vi "Crop Rotate Resize to U16.vi"() -> ()   [LabVIEW 2023]
uses:
  <vilib>/vision/NI_Vision_Development_Module.lvlib
panel:
  in  "2nd Resample":bool
  in  "2nd crop":bool
  in  "Symmetry":bool
  in  "Type of Symmetry":u32(ring)=1 items=["Horizontal", "Vertical", "Central", "1st Diagonal", "2nd Diagonal"]
  out "Image 3":T1(plugin-control)
  in  "Maintain Size":bool
  in  "resize":bool=TRUE
  in  "Do it":bool
  in  "stop":bool
  in  "Invert":bool
  in  "X Resolution":i32=1024
  in  "Y Resolution":i32=1024
  in  "Angle (degrees)":dbl format="%#_13g"
  in  "Destination File Path":path
  in  "Source File Path":path
  out "Image 2":T1(plugin-control)
  out "Image":T1(plugin-control)
  # "Nothing special, just my very internal VI to Crop/Resize/Rotate images if needed"
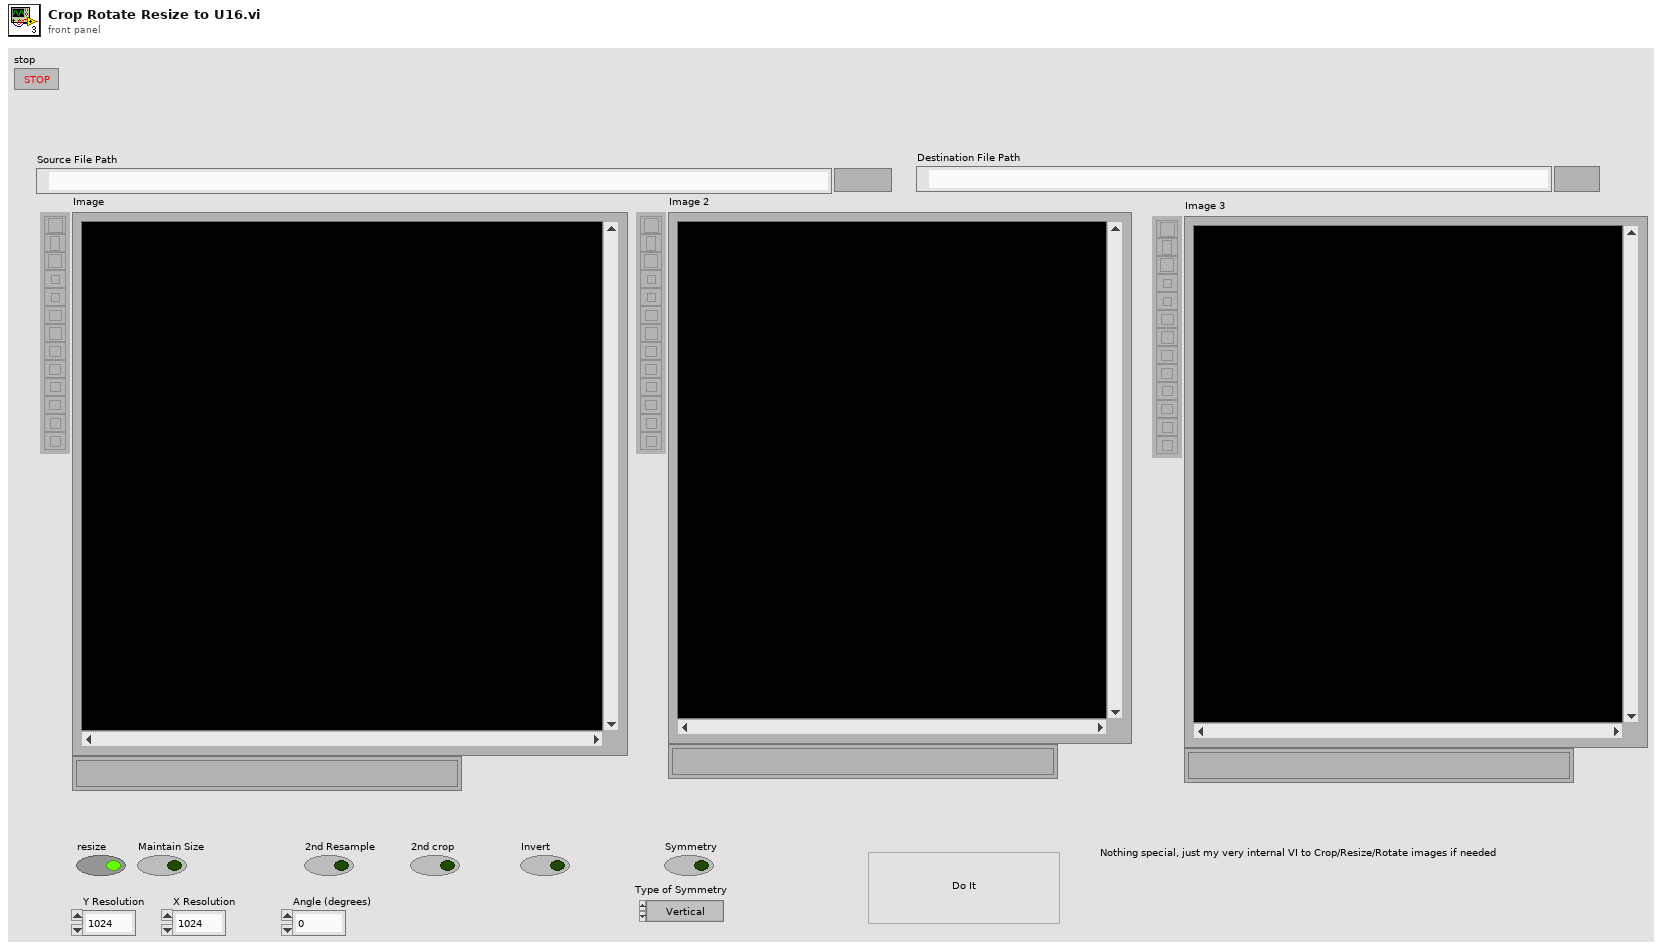
[diagram p1: front panel]
types:
  T1 = typedef "IMAQ Image.ctl" = refnum<image>
  T2 = typedef "Image Type" = u32
  T3 = cluster{"Global Rectangle":i32[], "Contours":cluster{"Contour Type":u32, "ROI Type":u32, "Points":i32[]}[]}
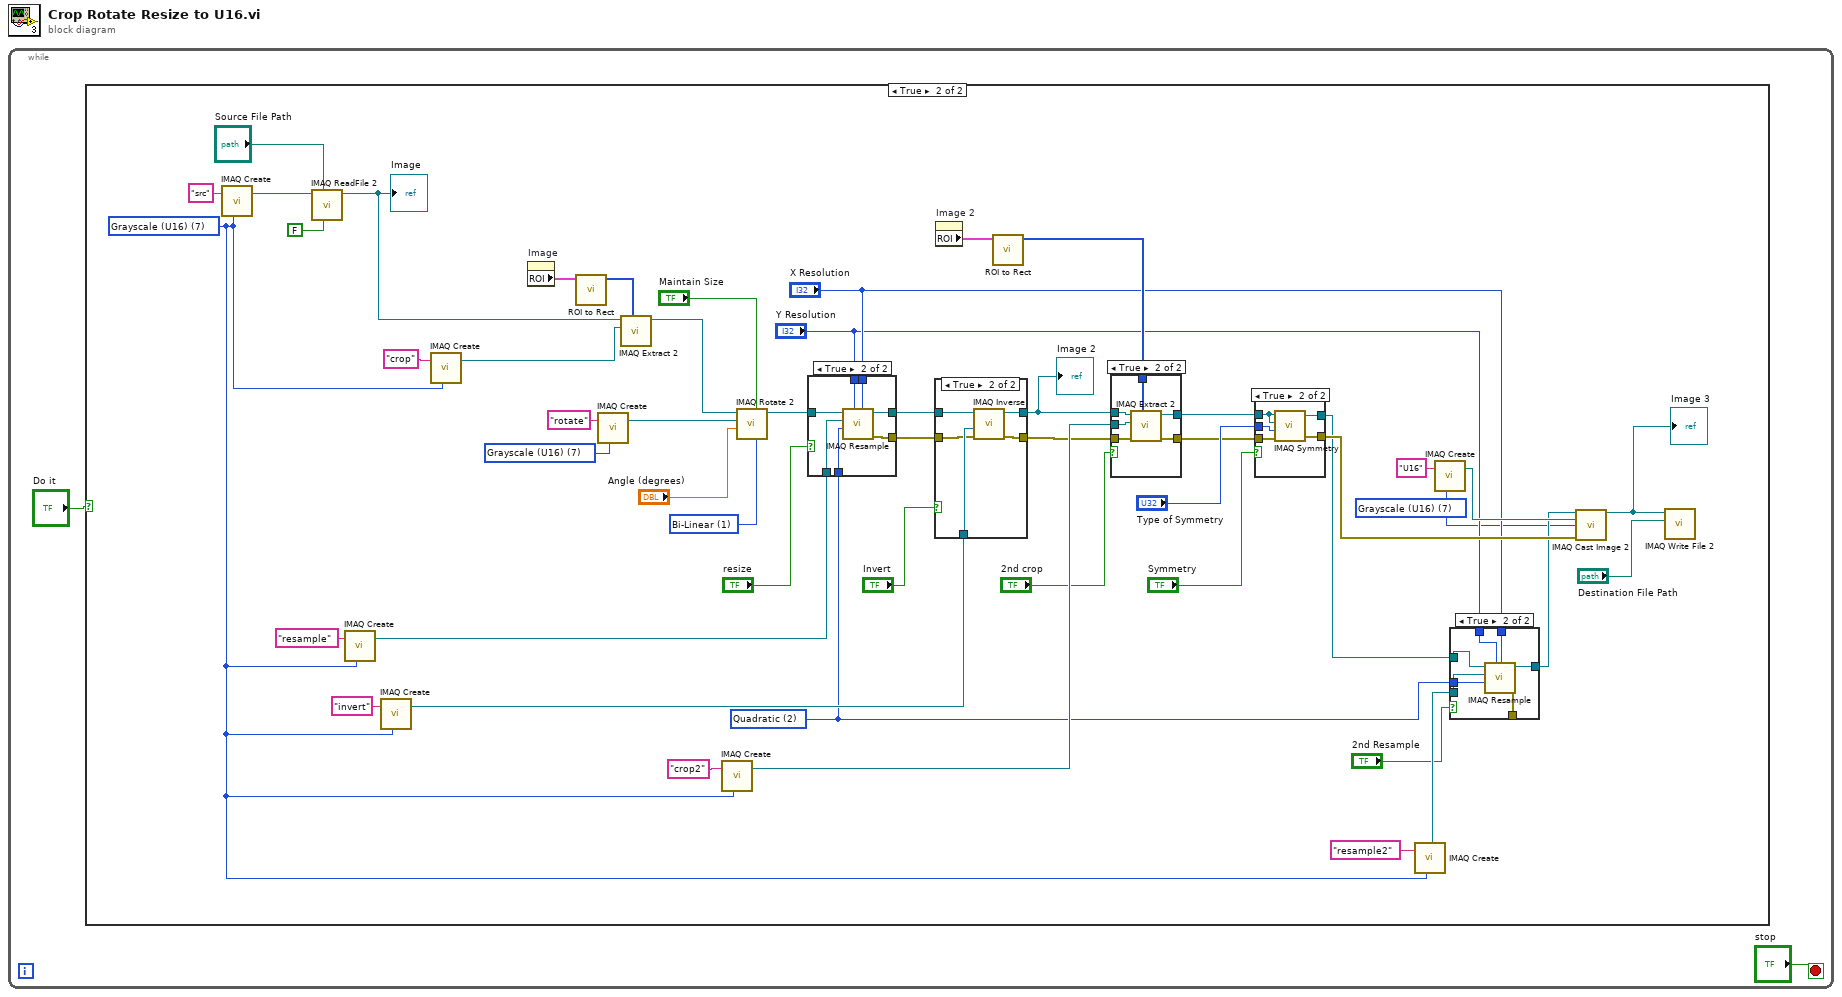
[diagram p0: block diagram]
diagram:
  n1 = while {
    stop <- "stop" stop-if-true
    n2 = case shown="True" "Do it" {
      frame False {
      }
      frame True {
        w3 = T2 7 items=["Grayscale (U8)", "Grayscale (I16)", "Grayscale (SGL)", "Complex (CSG)", "RGB (U32)", "HSL (U32)", "RGB (U64)", "Grayscale (U16)"] ("Image Type")
        w31 = 1 items=["Zero Order", "Bi-Linear"] ("Interpolation Type")
        w7 = u32 2 items=["Zero Order", "Bi-Linear", "Quadratic", "Cubic Spline"] ("Interpolation Type")
        w46 = T2 7 items=["Grayscale (U8)", "Grayscale (I16)", "Grayscale (SGL)", "Complex (CSG)", "RGB (U32)", "HSL (U32)", "RGB (U64)", "Grayscale (U16)"] ("Image Type")
        w6 = T2 7 items=["Grayscale (U8)", "Grayscale (I16)", "Grayscale (SGL)", "Complex (CSG)", "RGB (U32)", "HSL (U32)", "RGB (U64)", "Grayscale (U16)"] ("Image Type")
        n3 = call "IMAQ Create"("Image Name"="src", "Image Type"=w6) -> ("New Image"=w52:T1)  [unwired: 3 in, 1 out]
        n4 = call "IMAQ ReadFile 2"("Use File Path Image Type"=FALSE, "File Path"="Source File Path", "Image"=w52) -> ("Image Out"=w50:T1)  [unwired: 4 in, 4 out]
        "Image" <- w50
        n5 = call "IMAQ Create"("Image Name"="resample", "Image Type"=w6) -> ("New Image"=w39:T1)  [unwired: 3 in, 1 out]
        n6 = call "IMAQ Create"("Image Name"="invert", "Image Type"=w6) -> ("New Image"=w36:T1)  [unwired: 3 in, 1 out]
        n7 = call "IMAQ Create"("Image Name"="crop", "Image Type"=w6) -> ("New Image"=w48:T1)  [unwired: 3 in, 1 out]
        n8 = property on="Image" class="ImageControl"() -> ("ROI"=w5:T3)  [unwired: 2 in, 2 out]
        n9 = call "ROI to Rect.vi"("ROI"=w5) -> ("Rect"=w4:i32[])  [unwired: 9 in, 1 out]
        n10 = call "IMAQ Create"("Image Name"="rotate", "Image Type"=w46) -> ("New Image"=w44:T1)  [unwired: 3 in, 1 out]
        n11 = call "IMAQ Extract 2"("Optional Rectangle"=w4, "Image Dst"=w48, "Image Src"=w50) -> ("Image Dst Out"=w47:T1)  [unwired: 7 in, 1 out]
        n12 = call "IMAQ Create"("Image Name"="crop2", "Image Type"=w6) -> ("New Image"=w24:T1)  [unwired: 3 in, 1 out]
        n13 = call "IMAQ Rotate 2"("Interpolation Type"=w31, "Maintain Size"="Maintain Size", "Angle (degrees)"="Angle (degrees)", "Image Dst"=w44, "Image Src"=w47) -> ("Image Dst Out"=w41:T1)  [unwired: 5 in, 1 out]
        n14 = case shown="True" "resize" {
          tunnel: w41 -> [w76 w83]
          tunnel: w39 -> [_ w82]
          tunnel: "X Resolution" -> [_ w81]
          tunnel: "Y Resolution" -> [_ w80]
          tunnel: [w76 w79] -> w38
          tunnel: w7 -> [_ w78]
          tunnel: [_ w77] -> w19
          frame False {
          }
          frame True {
            n15 = call "IMAQ Resample"("X Resolution"=w81, "Y Resolution"=w80, "Interpolation Type"=w78, "Image Dst"=w82, "Image Src"=w83) -> ("error out"=w77:errorcluster, "Image Dst Out"=w79:T1)  [unwired: 5 in]
          }
        }
        n16 = case shown="True" "Invert" {
          tunnel: w38 -> [w84 w89]
          tunnel: w36 -> [_ w88]
          tunnel: [w84 w87] -> w26
          tunnel: w19 -> [_ w86]
          tunnel: [_ w85] -> w18
          frame False {
          }
          frame True {
            n17 = call "IMAQ Inverse"("error in (no error)"=w86, "Image Dst"=w88, "Image Src"=w89) -> ("error out"=w85:errorcluster, "Image Dst Out"=w87:T1)  [unwired: 7 in]
          }
        }
        "Image 2" <- w26
        n18 = property on="Image 2" class="ImageControl"() -> ("ROI"=w27:T3)  [unwired: 2 in, 2 out]
        n19 = call "ROI to Rect.vi"("ROI"=w27) -> ("Rect"=w28:i32[])  [unwired: 9 in, 1 out]
        n20 = case shown="True" "2nd crop" {
          tunnel: w28 -> [_ w69]
          tunnel: w26 -> [w63 w68]
          tunnel: w24 -> [_ w67]
          tunnel: [w63 w66] -> w22
          tunnel: w18 -> [w62 w65]
          tunnel: [w62 w64] -> w17
          frame False {
          }
          frame True {
            n21 = call "IMAQ Extract 2"("Optional Rectangle"=w69, "error in (no error)"=w65, "Image Dst"=w67, "Image Src"=w68) -> ("error out"=w64:errorcluster, "Image Dst Out"=w66:T1)  [unwired: 6 in]
          }
        }
        n22 = case shown="True" "Symmetry" {
          tunnel: [w70 w75] -> w14
          tunnel: w22 -> [w70 w74]
          tunnel: "Type of Symmetry" -> [_ w73]
          tunnel: w17 -> [_ w72]
          tunnel: [_ w71] -> w16
          frame False {
          }
          frame True {
            n23 = call "IMAQ Symmetry"("error in (no error)"=w72, "Type of Symmetry"=w73, "Image Dst"=w74, "Image Src"=w74) -> ("error out"=w71:errorcluster, "Image Dst Out"=w75:T1)  [unwired: 1 in]
          }
        }
        n24 = call "IMAQ Create"("Image Name"="resample2", "Image Type"=w6) -> ("New Image"=w11:T1)  [unwired: 3 in, 1 out]
        n25 = call "IMAQ Create"("Image Name"="U16", "Image Type"=w3) -> ("New Image"=w34:T1)  [unwired: 3 in, 1 out]
        n26 = case shown="True" "2nd Resample" {
          tunnel: w14 -> [w54 w61]
          tunnel: w11 -> [_ w60]
          tunnel: [w54 w59] -> w13
          tunnel: [_ w58] -> _
          tunnel: "X Resolution" -> [_ w57]
          tunnel: "Y Resolution" -> [_ w56]
          tunnel: w7 -> [_ w55]
          frame False {
          }
          frame True {
            n27 = call "IMAQ Resample"("X Resolution"=w57, "Y Resolution"=w56, "Interpolation Type"=w55, "Image Dst"=w60, "Image Src"=w61) -> ("error out"=w58:errorcluster, "Image Dst Out"=w59:T1)  [unwired: 5 in]
          }
        }
        n28 = call "IMAQ Cast Image 2"("Image Src"=w13, "Image Dst"=w34, "Image Type"=w3, "error in (no error)"=w16) -> ("Image Dst Out"=w23:T1)  [unwired: 10 in, 1 out]
        "Image 3" <- w23
        n29 = call-poly "IMAQ Write File 2"("File Path"="Destination File Path", "Image"=w23) -> ()  [unwired: 8 in, 2 out]
      }
    }
  }
